vi "Start Acquisition.vi"(8 "error in (no error)":errorcluster, 10 "Camera State In":T3 {"Sub Region"."V Size"."Value" min=0 max=0 step=4; "Sub Region"."H Size"."Value" min=0 max=0 step=4; "Sub Region"."V Offset"."Value" min=0 max=0 step=4; "Sub Region"."H Offset"."Value" min=0 max=0 step=4}, 11 "Acquisition Settings":T1={"Save?"=FALSE, "DCIMG Path"=path "E:/test2", "Filename"="test", "Total Frames"=15, "Sender"=enum."UI"}) -> (0 "error out":errorcluster {"code" format="%.0x"}, 1 "New Image Out":T2, 2 "Camera State Out":T3 {"Sub Region"."V Size"."Value" min=0 max=0 step=4; "Sub Region"."H Size"."Value" min=0 max=0 step=4; "Sub Region"."V Offset"."Value" min=0 max=0 step=4; "Sub Region"."H Offset"."Value" min=0 max=0 step=4})   [LabVIEW 2015]
uses:
  Camera State.ctl
  Camera Loop State.ctl
  <vilib>/Utility/miscctls.llb/LVMinMaxIncTypeDef.ctl
  Acquisition Settings.ctl
  Live View State.ctl
  <vilib>/vision/Image Controls.llb/IMAQ Image.ctl
  Camera.lvlib
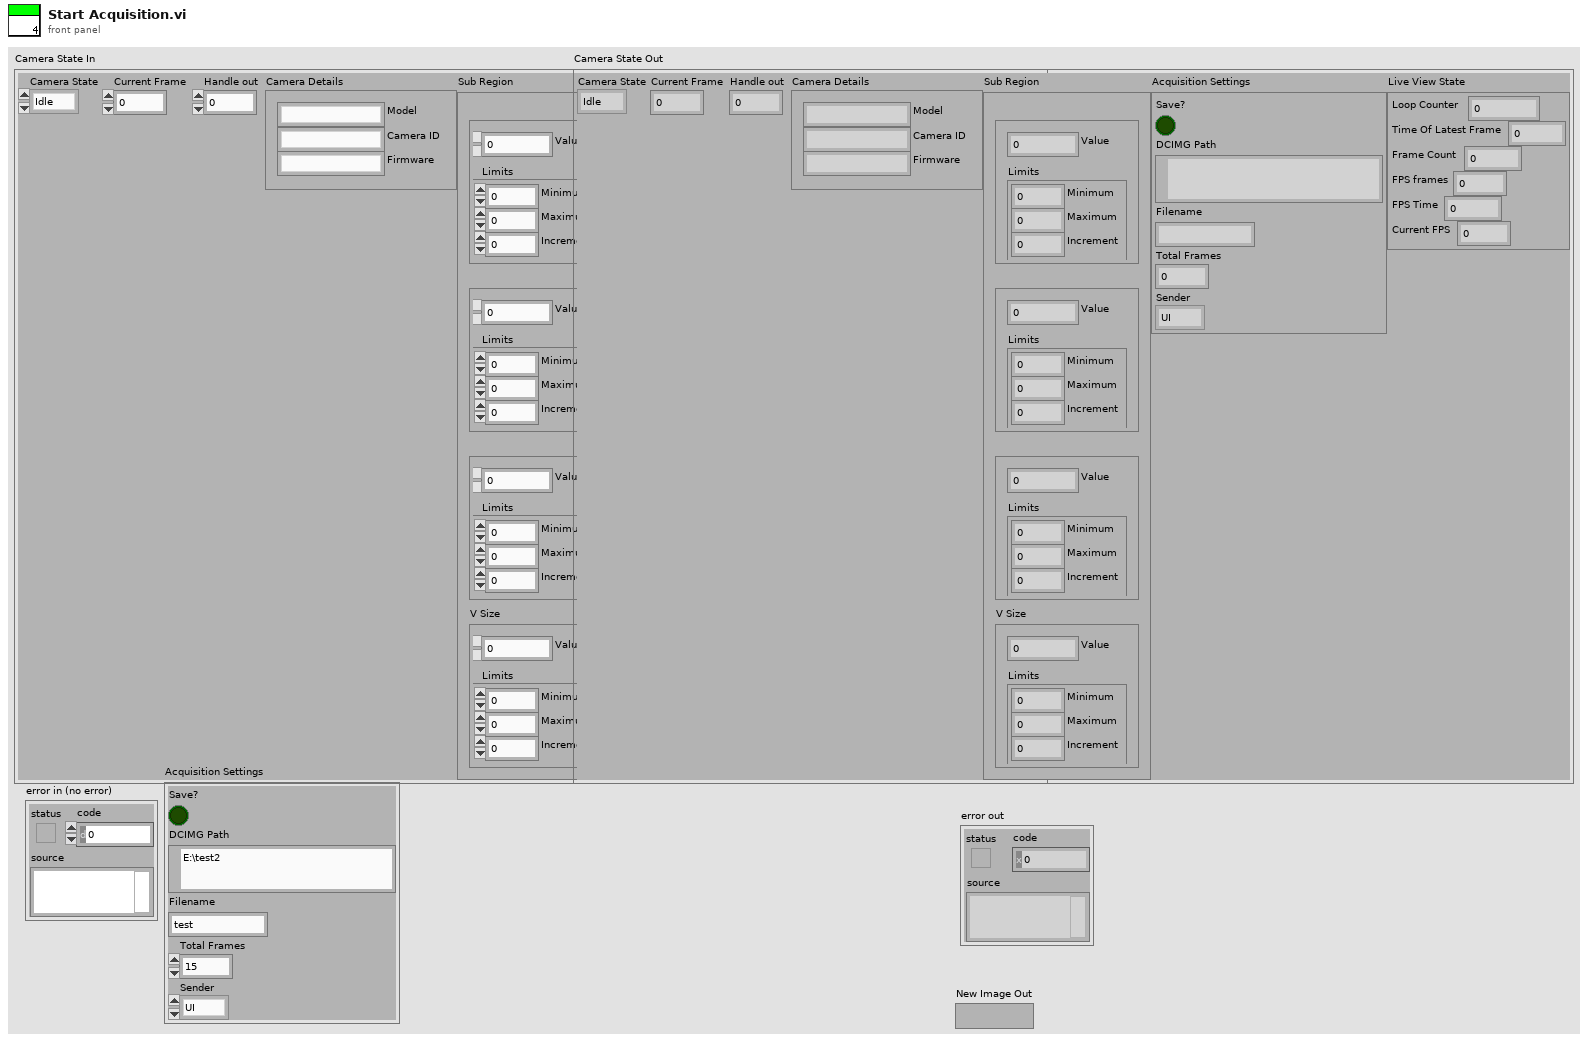
[diagram p1: front panel]
types:
  T1 = typedef "Camera.lvlib/Acquisition Settings.ctl" = cluster{"Save?":bool, "DCIMG Path":path, "Filename":string, "Total Frames":i32, "Sender":enum16{"UI", "Automation"}}
  T2 = typedef "IMAQ Image.ctl" = refnum<image>
  T3 = typedef "Camera.lvlib/Camera State.ctl" = cluster{"Camera State":T4, "Current Frame":i32, "Handle out":u32, "Camera Details":cluster{"Model":string, "Camera ID":string, "Firmware":string}, "Sub Region":cluster{"H Offset":cluster{"Value":i32, "Limits":T5}, "V Offset":cluster{"Value":i32, "Limits":T5}, "H Size":cluster{"Value":i32, "Limits":T5}, "V Size":cluster{"Value":i32, "Limits":T5}}, "Acquisition Settings":T1, "Live View State":T6}
  T4 = typedef "Camera.lvlib/Camera Loop State.ctl" = enum16{"Idle", "Live View", "Ready", "Acquiring"}
  T5 = typedef "LVMinMaxIncTypeDef.ctl" = cluster{"Minimum":dbl, "Maximum":dbl, "Increment":dbl}
  T6 = typedef "Camera.lvlib/Live View State.ctl" = cluster{"Loop Counter":i32, "Time Of Latest Frame":u32, "Frame Count":u32, "FPS frames":dbl, "FPS Time":u32, "Current FPS":dbl}
  T7 = cluster{"Mode":u32, "Polarity":u32, "Times":u32, "Delay":dbl}
  T8 = cluster{"H Offset":cluster{"Value":i32, "Limits":T5}, "V Offset":cluster{"Value":i32, "Limits":T5}, "H Size":cluster{"Value":i32, "Limits":T5}, "V Size":cluster{"Value":i32, "Limits":T5}}
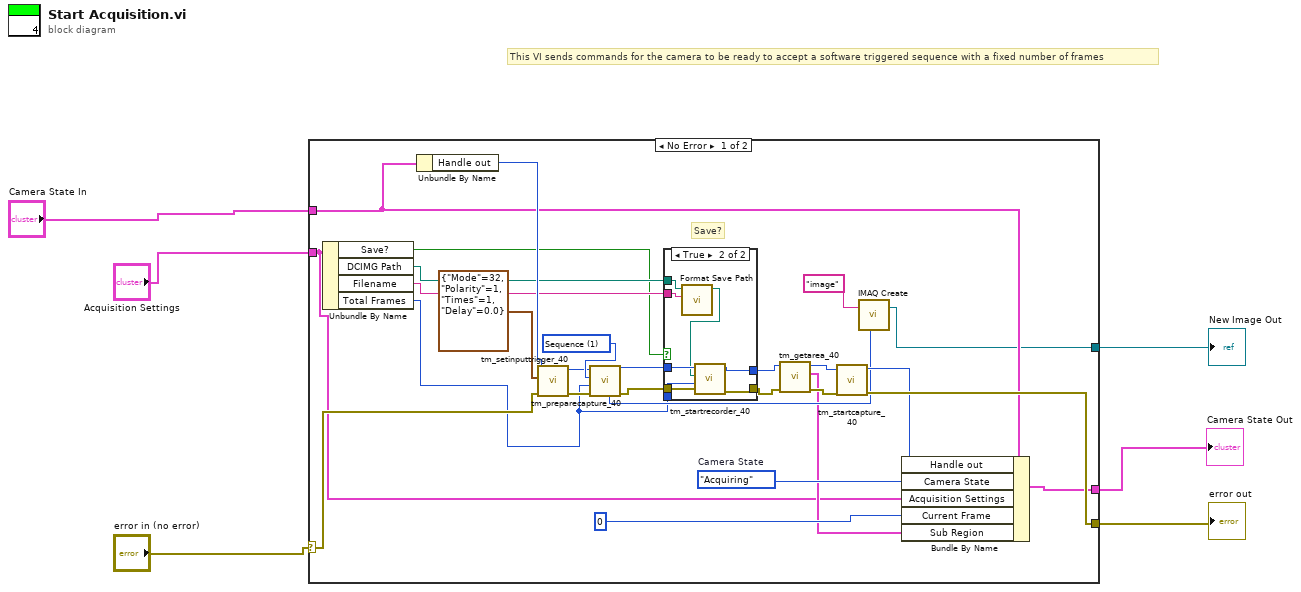
[diagram p0: block diagram]
diagram:
  # "This VI sends commands for the camera to be ready to accept a software triggered sequence with a fixed number of frames"
  n1 = case shown="No Error" "error in (no error)" {
    selector: "error in (no error)" -> [w21 w45]
    tunnel: [w26 w45] -> w6
    tunnel: "Camera State In" -> [w20 w44]
    tunnel: [w22 w44] -> w4
    tunnel: [w19 _] -> w2
    tunnel: "Acquisition Settings" -> [w7 _]
    frame No Error {
      w28 = Camera_Loop_State."Acquiring"  # Camera State
      w33 = 1 items=["Snap", "Sequence"] ("Capture mode")
      # "Save?"
      n2 = Unbundle By Name(w7) -> ("Save?"=w8:bool, "DCIMG Path"=w9:path, "Filename"=w10:string, "Total Frames"=w11:i32)
      n3 = Unbundle By Name(w20) -> ("Handle out"=w29:u32)
      n4 = call <userlib>:"tm_setinputtrigger_40.vi"("error in (no error)"=w21, "Parameters"=T7 {"Mode"=32, "Polarity"=1, "Times"=1, "Delay"=0.0}, "Handle in"=w29) -> ("error out"=w31:errorcluster, "Handle out"=w32:u32)  [unwired: 7 in]
      n5 = call <userlib>:"tm_preparecapture_40.vi"("error in (no error)"=w31, "Frames"=w11, "Capture mode"=w33, "Handle in"=w32) -> ("error out"=w12:errorcluster, "Handle out"=w14:u32, "Image type"=w23:u32)  [unwired: 4 in, 1 out]
      n6 = case shown="True" w8 {
        tunnel: [w35 w43] -> w15
        tunnel: w14 -> [w35 w42]
        tunnel: [w34 w41] -> w13
        tunnel: w12 -> [w34 w40]
        tunnel: w11 -> [_ w38]
        tunnel: w10 -> [_ w37]
        tunnel: w9 -> [_ w36]
        frame False {
        }
        frame True {
          n7 = call "Format Save Path.vi"("Filename"=w37, "DCIMG Path"=w36) -> ("appended path"=w39:path)  [unwired: 9 in]
          n8 = call <userlib>:"tm_startrecorder_40.vi"("error in (no error)"=w40, "frames"=w38, "File"=w39, "Handle in"=w42) -> ("error out"=w41:errorcluster, "Handle out"=w43:u32)  [unwired: 6 in]
        }
      }
      n9 = call <userlib>:"tm_getarea_40.vi"("error in (no error)"=w13, "Handle in"=w15) -> ("error out"=w17:errorcluster, "Sub Region"=w16:T8, "Handle out"=w18:u32)  [unwired: 7 in]
      n10 = call <userlib>:"tm_startcapture_40.vi"("error in (no error)"=w17, "Handle in"=w18) -> ("error out"=w26:errorcluster, "Handle out"=w25:u32)  [unwired: 8 in]
      n11 = call "IMAQ Create"("Image Name"="image", "Image Type"=w23) -> ("New Image"=w19:T2)  [unwired: 3 in, 1 out]
      n12 = Bundle By Name(cluster=w20, "Handle out"=w25, "Camera State"=w28, "Acquisition Settings"=w7, "Current Frame"=0, "Sub Region"=w16) -> (w22:T3)
    }
    frame Error {
    }
  }
  "Camera State Out" <- w4
  "error out" <- w6
  "New Image Out" <- w2
